vi "IntakeDisable.vi"   [LabVIEW 2014, in "IntakeLib.lvlib"]
uses:
  IntakeLib.lvlib
  IntakeRefs.ctl
types:
  T1 = typedef "IntakeLib.lvlib/IntakeRefs.ctl" = enum16{"FrontRightIntakeMotor", "FrontLeftIntakeMotor", "BackLeftIntakeMotor", "BackRightIntakeMotor"}
  T2 = typedef "WPI_MotorControlDeviceRef.ctl" = cluster{"DeviceStatus":errorcluster, "Type":T3, "PWM":cluster{"Controller":T4, "PWM Channel":T5, "DeadBand":T6}, "CAN":cluster{"Device Number":u8, "Control Mode":T7, "Semaphore":T8, "Max Vout":dbl, "TalonSRX Control Mode":T9}, "Invert":bool, "TransformRef":T10, "InvTransformRef":T10}
  T3 = typedef "WPI_MotorControlType.ctl" = enum16{"PWM", "CAN", "CANTalonSRX"}
  T4 = typedef "FPGA_TypedefDigitalModule.ctl" = enum16{"Controller 1"}
  T5 = typedef "FPGA_DIOPWMChannel.ctl" = enum8{"PWM 0", "PWM 1", "PWM 2", "PWM 3", "PWM 4", "PWM 5", "PWM 6", "PWM 7", "PWM 8", "PWM 9", "PWM MXP 0", "PWM MXP 1", "PWM MXP 2", "PWM MXP 3", "PWM MXP 4", "PWM MXP 5", "PWM MXP 6", "PWM MXP 7", "PWM MXP 8", "PWM MXP 9", "Invalid"}
  T6 = typedef "WPI_PWMDeadband.ctl" = cluster{"Name":string, "maxPositivePwm":i32, "minPositivePwm":i32, "centerPwm":i32, "maxNegativePwm":i32, "minNegativePwm":i32, "angularRange":u16}
  T7 = typedef "WPI_CANJaguar_ControlMode.ctl" = enum8{"Percent VBus", "Current", "Speed", "Position", "Voltage"}
  T8 = typedef "Semaphore RefNum" = refnum<k1>
  T9 = typedef "WPI_CANTalonSRX_APIControlMode.ctl" = enum8{"Percent VBus", "Speed", "Position", "Slave", "Unchanged / Invalid"}
  T10 = typedef "WPI_PWMTransform_ConPane.ctl" = refnum<vi>
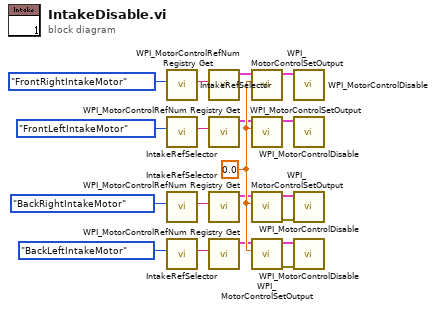
[diagram p0: block diagram]
diagram:
  w11 = 0.0 ("Output")
  n1 = call "IntakeRefSelector.vi"("Enum 2"=IntakeRefs."FrontRightIntakeMotor") -> ("String"=w12:string)  [unwired: 10 in]
  n2 = call "IntakeRefSelector.vi"("Enum 2"=IntakeRefs."FrontLeftIntakeMotor") -> ("String"=w13:string)  [unwired: 10 in]
  n3 = call "IntakeRefSelector.vi"("Enum 2"=IntakeRefs."BackRightIntakeMotor") -> ("String"=w14:string)  [unwired: 10 in]
  n4 = call "IntakeRefSelector.vi"("Enum 2"=IntakeRefs."BackLeftIntakeMotor") -> ("String"=w15:string)  [unwired: 10 in]
  n5 = call <vilib>:"WPI_MotorControlRefNum Registry Get.vi"("refnum name"=w12) -> ("MotorControlDevRef"=w10:T2)  [unwired: 9 in, 1 out]
  n6 = call <vilib>:"WPI_MotorControlRefNum Registry Get.vi"("refnum name"=w13) -> ("MotorControlDevRef"=w9:T2)  [unwired: 9 in, 1 out]
  n7 = call <vilib>:"WPI_MotorControlRefNum Registry Get.vi"("refnum name"=w14) -> ("MotorControlDevRef"=w8:T2)  [unwired: 9 in, 1 out]
  n8 = call <vilib>:"WPI_MotorControlRefNum Registry Get.vi"("refnum name"=w15) -> ("MotorControlDevRef"=w7:T2)  [unwired: 9 in, 1 out]
  n9 = call <vilib>:"WPI_MotorControlSetOutput.vi"("Output"=w11, "MotorControlDevRef"=w10) -> ("MotorControlDevRef"=w6:T2)  [unwired: 7 in, 2 out]
  n10 = call <vilib>:"WPI_MotorControlSetOutput.vi"("Output"=w11, "MotorControlDevRef"=w9) -> ("MotorControlDevRef"=w5:T2)  [unwired: 7 in, 2 out]
  n11 = call <vilib>:"WPI_MotorControlSetOutput.vi"("Output"=w11, "MotorControlDevRef"=w8) -> ("error out"=w4:errorcluster, "MotorControlDevRef"=w3:T2)  [unwired: 7 in, 1 out]
  n12 = call <vilib>:"WPI_MotorControlSetOutput.vi"("Output"=w11, "MotorControlDevRef"=w7) -> ("error out"=w2:errorcluster, "MotorControlDevRef"=w1:T2)  [unwired: 7 in, 1 out]
  n13 = call <vilib>:"WPI_MotorControlDisable.vi"("MotorControlDevRef"=w6) -> ()  [unwired: 9 in, 2 out]
  n14 = call <vilib>:"WPI_MotorControlDisable.vi"("MotorControlDevRef"=w5) -> ()  [unwired: 9 in, 2 out]
  n15 = call <vilib>:"WPI_MotorControlDisable.vi"("error in (no error)"=w4, "MotorControlDevRef"=w3) -> ()  [unwired: 8 in, 2 out]
  n16 = call <vilib>:"WPI_MotorControlDisable.vi"("error in (no error)"=w2, "MotorControlDevRef"=w1) -> ()  [unwired: 8 in, 2 out]
